vi "Lab Panel V5.29.vi"() -> ()   [LabVIEW 2013] (continued)
                    n2198 = Multiply(x=w3863, y=w3857) -> (x*y=w3850:dbl)
                    n2199 = Multiply(x=w3862, y=w3856) -> (x*y=w3849:dbl)
                    n2200 = Multiply(x=w3861, y=w3855) -> (x*y=w3848:dbl)
                    n2201 = Multiply(x=w3860, y=w3854) -> (x*y=w3846:dbl)
                    n2202 = Multiply(x=w3859, y=w3853) -> (x*y=w3845:dbl)
                    n2203 = Multiply(x=w3858, y=w3852) -> (x*y=w3844:dbl)
                    n2204 = local read "SIG LAB02-1"() -> (w3851:T2)
                    n2205 = local read "SIG LAB02-2"() -> (w3847:T2)
                    n2206 = Bundle By Name(cluster=w3851, "AMPS"=w3850, "VOLTS"=w3849, "PF"=w3848) -> (w3843:T2)
                    n2207 = Bundle By Name(cluster=w3847, "AMPS"=w3846, "VOLTS"=w3845, "PF"=w3844) -> (w3842:T2)
                    n2208 = global write "Global display 1.vi" "SIG LAB02-1"(w3843) -> ()
                    n2209 = local write "SIG LAB02-2"(w3842) -> ()
                    n2210 = global write "Global display 1.vi" "SIG LAB02-2"(w3842) -> ()
                    n2211 = local write "SIG LAB02-1"(w3843) -> ()
                  }
                  frame #4 {
                    n2212 = Unbundle By Name(w3895) -> ("OFF amps"=w3891:dbl, "VOLTS"=w3890:dbl, "PF"=w3889:dbl, "OFF amps"=w3888:dbl, "VOLTS"=w3887:dbl, "PF"=w3886:dbl)
                    n2213 = case shown="True" w3894 {
                      tunnel: [w3896 w3897] -> w3892
                      tunnel: w3893 -> [_ w3897]
                      frame False {
                        n2214 = local read "CAL LAB03"() -> (w3896:T14)
                      }
                      frame True {
                      }
                    }
                    n2215 = Unbundle By Name(w3892) -> ("1  (A) cal"=w3885:dbl, "1 (V) cal"=w3884:dbl, "1 (PF) cal"=w3883:dbl, "2 (A) cal"=w3882:dbl, "2 (V) cal"=w3881:dbl, "2 (PF) cal"=w3880:dbl)  [unwired: 4 out]
                    n2216 = Multiply(x=w3891, y=w3885) -> (x*y=w3878:dbl)
                    n2217 = Multiply(x=w3890, y=w3884) -> (x*y=w3872:dbl)
                    n2218 = Multiply(x=w3889, y=w3883) -> (x*y=w3877:dbl)
                    n2219 = Multiply(x=w3888, y=w3882) -> (x*y=w3875:dbl)
                    n2220 = Multiply(x=w3887, y=w3881) -> (x*y=w3874:dbl)
                    n2221 = Multiply(x=w3886, y=w3880) -> (x*y=w3873:dbl)
                    n2222 = local read "SIG LAB03-1"() -> (w3879:T2)
                    n2223 = local read "SIG LAB03-2"() -> (w3876:T2)
                    n2224 = Bundle By Name(cluster=w3879, "AMPS"=w3878, "VOLTS"=w3872, "PF"=w3877) -> (w3871:T2)
                    n2225 = Bundle By Name(cluster=w3876, "AMPS"=w3875, "VOLTS"=w3874, "PF"=w3873) -> (w3870:T2)
                    n2226 = global write "Global display 1.vi" "SIG LAB03-1"(w3871) -> ()
                    n2227 = global write "Global display 1.vi" "SIG LAB03-2"(w3870) -> ()
                    n2228 = local write "SIG LAB03-2"(w3870) -> ()
                    n2229 = local write "SIG LAB03-1"(w3871) -> ()
                  }
                  frame #5 {
                    n2230 = case shown="False" w3922 {
                      tunnel: [w3924 w3925] -> w3920
                      tunnel: w3921 -> [_ w3925]
                      frame False {
                        n2231 = local read "CAL LAB04"() -> (w3924:T14)
                      }
                      frame True {
                      }
                    }
                    n2232 = Unbundle By Name(w3923) -> ("OFF amps"=w3919:dbl, "VOLTS"=w3918:dbl, "PF"=w3917:dbl, "OFF amps"=w3916:dbl, "VOLTS"=w3915:dbl, "PF"=w3914:dbl)
                    n2233 = Unbundle By Name(w3920) -> ("1  (A) cal"=w3913:dbl, "1 (V) cal"=w3912:dbl, "1 (PF) cal"=w3911:dbl, "2 (A) cal"=w3910:dbl, "2 (V) cal"=w3909:dbl, "2 (PF) cal"=w3908:dbl)  [unwired: 4 out]
                    n2234 = Multiply(x=w3919, y=w3913) -> (x*y=w3906:dbl)
                    n2235 = Multiply(x=w3918, y=w3912) -> (x*y=w3905:dbl)
                    n2236 = Multiply(x=w3917, y=w3911) -> (x*y=w3904:dbl)
                    n2237 = Multiply(x=w3916, y=w3910) -> (x*y=w3902:dbl)
                    n2238 = Multiply(x=w3915, y=w3909) -> (x*y=w3901:dbl)
                    n2239 = Multiply(x=w3914, y=w3908) -> (x*y=w3900:dbl)
                    n2240 = local read "SIG LAB04-1"() -> (w3907:T2)
                    n2241 = local read "SIG LAB04-2"() -> (w3903:T2)
                    n2242 = Bundle By Name(cluster=w3907, "AMPS"=w3906, "VOLTS"=w3905, "PF"=w3904) -> (w3899:T2)
                    n2243 = Bundle By Name(cluster=w3903, "AMPS"=w3902, "VOLTS"=w3901, "PF"=w3900) -> (w3898:T2)
                    n2244 = global write "Global display 1.vi" "SIG LAB04-2"(w3898) -> ()
                    n2245 = global write "Global display 1.vi" "SIG LAB04-1"(w3899) -> ()
                    n2246 = local write "SIG LAB04-2"(w3898) -> ()
                    n2247 = local write "SIG LAB04-1"(w3899) -> ()
                  }
                  frame #6 {
                    n2248 = Unbundle By Name(w3951) -> ("OFF amps"=w3947:dbl, "VOLTS"=w3928:dbl, "PF"=w3946:dbl, "OFF amps"=w3945:dbl, "VOLTS"=w3944:dbl, "PF"=w3943:dbl)
                    n2249 = case shown="False" w3950 {
                      tunnel: [w3952 w3953] -> w3948
                      tunnel: w3949 -> [_ w3953]
                      frame False {
                        n2250 = local read "CAL LAB05"() -> (w3952:T14)
                      }
                      frame True {
                      }
                    }
                    n2251 = Unbundle By Name(w3948) -> ("1  (A) cal"=w3942:dbl, "1 (V) cal"=w3941:dbl, "1 (PF) cal"=w3940:dbl, "2 (A) cal"=w3939:dbl, "2 (V) cal"=w3938:dbl, "2 (PF) cal"=w3937:dbl)  [unwired: 4 out]
                    n2252 = Multiply(x=w3947, y=w3942) -> (x*y=w3935:dbl)
                    n2253 = Multiply(x=w3928, y=w3941) -> (x*y=w3934:dbl)
                    n2254 = Multiply(x=w3946, y=w3940) -> (x*y=w3933:dbl)
                    n2255 = Multiply(x=w3945, y=w3939) -> (x*y=w3931:dbl)
                    n2256 = Multiply(x=w3944, y=w3938) -> (x*y=w3930:dbl)
                    n2257 = Multiply(x=w3943, y=w3937) -> (x*y=w3929:dbl)
                    n2258 = local read "SIG LAB05-1"() -> (w3936:T2)
                    n2259 = local read "SIG LAB05-2"() -> (w3932:T2)
                    n2260 = Bundle By Name(cluster=w3936, "AMPS"=w3935, "VOLTS"=w3934, "PF"=w3933) -> (w3927:T2)
                    n2261 = Bundle By Name(cluster=w3932, "AMPS"=w3931, "VOLTS"=w3930, "PF"=w3929) -> (w3926:T2)
                    n2262 = global write "Global display 1.vi" "SIG LAB05-1"(w3927) -> ()
                    n2263 = global write "Global display 1.vi" "SIG LAB05-2"(w3926) -> ()
                    n2264 = local write "SIG LAB05-2"(w3926) -> ()
                    n2265 = local write "SIG LAB05-1"(w3927) -> ()
                  }
                  frame #7 {
                    n2266 = case shown="False" w3954 {
                      tunnel: w3956 -> [w3961 _]
                      tunnel: w3955 -> [w3960 _]
                      frame False {
                        # "update ambient referance temperature"
                        n2267 = case shown="True" w3961 {
                          tunnel: [w3963 100.0] -> w3962
                          frame False {
                            n2268 = local read "TEMP REF cal"() -> (w3963:dbl)
                          }
                          frame True {
                          }
                        }
                        n2269 = disable-structure shown="Disabled" {
                          frame Disabled {
                            n2270 = local read "Temp read loop"() -> ()  [unwired: 1 out]
                          }
                          frame Enabled {
                          }
                        }
                        n2271 = Multiply(x=w3962, y=w3960) -> (x*y=w3959:dbl)
                        n2272 = Subtract(x=w3959, y=272) -> (x-y=w3957:dbl)
                        "Amb Tp" <- w3957
                        n2273 = local write "Ref deg C"(w3957) -> ()
                        "deg C (volts)" <- w3960
                      }
                      frame True {
                      }
                    }
                  }
                }
              }
            }
          }
          frame #14 {
            # "save test data to file during testing"
            n2274 = local read "on loops"() -> (w3984:dbl)
            n2275 = Get Date/Time In Seconds() -> (seconds since 1Jan1904=w3965:timestamp)
            "File Time Stamp" <- w3965
            n2276 = local read "jig cycle"() -> (w3981:dbl)
            n2277 = Format Date/Time String(time format string (%c)="%H:%M%:%S", seconds (now)=w3965) -> (date/time string=w3969:string)  [unwired: 1 in]
            n2278 = Add(x=w3984, y=4) -> (x+y=w3982:dbl)
            n2279 = Build Array(w3969) -> (w3968:string[])
            n2280 = Equal?(x=w3981, y=3) -> (x = y?=w3967:bool)
            n2281 = Equal?(x=w3981, y=w3982) -> (x = y?=w3966:bool)
            n2282 = stacked-sequence {
              tunnel: w3980 -> [w3990 _ _ _ _ _ _ _ _ _]
              tunnel: w3979 -> [_ w4066 _ _ _ _ _ _ _ _]
              tunnel: w3978 -> [_ _ w4146 _ _ _ _ _ _ _]
              tunnel: w3977 -> [_ _ _ w4226 _ _ _ _ _ _]
              tunnel: w3976 -> [_ _ _ _ w4306 _ _ _ _ _]
              tunnel: w3975 -> [_ _ _ _ _ w4386 _ _ _ _]
              tunnel: w3974 -> [_ _ _ _ _ _ w4466 _ _ _]
              tunnel: w3973 -> [_ _ _ _ _ _ _ w4546 _ _]
              tunnel: w3972 -> [_ _ _ _ _ _ _ _ w4626 _]
              tunnel: w3971 -> [_ _ _ _ _ _ _ _ _ w4706]
              tunnel: w3968 -> [w3989 w4070 w4150 w4230 w4310 w4390 w4470 w4550 w4630 w4710]
              tunnel: w3967 -> [w3988 w4069 w4149 w4229 w4309 w4389 w4469 w4549 w4629 w4709]
              tunnel: w3966 -> [w3987 w4068 w4148 w4228 w4308 w4388 w4468 w4548 w4628 w4708]
              tunnel: w3965 -> [w3986 w4067 w4147 w4227 w4307 w4387 w4467 w4547 w4627 w4707]
              frame #0 {
                n2283 = case shown="True" w3990 {
                  tunnel: w3989 -> [_ w3995]
                  tunnel: w3988 -> [_ w3994]
                  tunnel: w3987 -> [_ w3992]
                  tunnel: w3986 -> [_ w3991]
                  frame False {
                  }
                  frame True {
                    n2284 = local read "DISP LAB01-1"() -> (w3996:T4)
                    n2285 = local read "SIG LAB01-1"() -> (w3997:T2)
                    n2286 = local read "ON L01-1"() -> (w3993:cluster{"amps":dbl, "volts":dbl, "pf":dbl})
                    n2287 = Unbundle(w3997) -> ("AMPS"=w4003:dbl, "VOLTS"=w4001:dbl, "PF"=w4000:dbl, "Tmp Live"=w3999:dbl, "Tmp Neut"=w4002:dbl)
                    n2288 = Unbundle(w3996) -> ("CYCLE"=w3998:dbl)  [unwired: 2 out]
                    n2289 = stacked-sequence {
                      tunnel: w4003 -> [w4007 w4026]
                      tunnel: w4002 -> [_ w4025]
                      tunnel: w4001 -> [w4006 w4024]
                      tunnel: w4000 -> [w4005 w4023]
                      tunnel: w3999 -> [_ w4022]
                      tunnel: w3998 -> [_ w4021]
                      tunnel: w3995 -> [_ w4020]
                      tunnel: w3994 -> [w4008 _]
                      tunnel: w3993 -> [w4004 w4018]
                      tunnel: w3992 -> [_ w4019]
                      tunnel: w3991 -> [_ w4014]
                      frame #0 {
                        n2290 = case shown="True" w4008 {
                          tunnel: w4007 -> [_ w4013]
                          tunnel: w4006 -> [_ w4012]
                          tunnel: w4005 -> [_ w4011]
                          tunnel: w4004 -> [_ w4009]
                          frame False {
                          }
                          frame True {
                            n2291 = Bundle(cluster=w4009, "amps"=w4013, "volts"=w4012, "pf"=w4011) -> (w4010:cluster{"amps":dbl, "volts":dbl, "pf":dbl})
                            n2292 = local write "ON L01-1"(w4010) -> ()
                          }
                        }
                      }
                      frame #1 {
                        n2293 = Unbundle(w4018) -> ("amps"=w4017:dbl, "volts"=w4016:dbl, "pf"=w4015:dbl)
                        n2294 = case shown="True" w4019 {
                          tunnel: w4026 -> [_ w4027]
                          tunnel: w4025 -> [_ w4065]
                          tunnel: w4024 -> [_ _]
                          tunnel: w4023 -> [_ _]
                          tunnel: w4022 -> [_ w4064]
                          tunnel: w4021 -> [_ w4063]
                          tunnel: w4020 -> [_ w4031]
                          tunnel: w4017 -> [_ w4028]
                          tunnel: w4016 -> [_ w4060]
                          tunnel: w4015 -> [_ w4059]
                          tunnel: w4014 -> [_ w4029]
                          frame False {
                          }
                          frame True {
                            n2295 = local read "TDMS LAB01-1"() -> (w4062:refnum<k34>)
                            n2296 = Build Array(w4060) -> (w4056:dbl[])
                            n2297 = Build Array(w4059) -> (w4055:dbl[])
                            n2298 = Build Array(w4064) -> (w4054:dbl[])
                            n2299 = Build Array(w4065) -> (w4053:dbl[])
                            n2300 = Build Array(w4028) -> (w4058:dbl[])
                            n2301 = Build Array(w4027) -> (w4057:dbl[])
                            n2302 = Build Array(w4063) -> (w4052:dbl[])
                            n2303 = Build Array("AMPS ON", "AMPS OFF", "VOLTS", "PF", "TEMP Live", "TEMP Neut", "CYCLE") -> (w4036:string[])
                            n2304 = Bundle By Name("Y"=w4058, "t0"=w4029) -> (w4051:waveform(dbl))  [unwired: 1 in]
                            n2305 = Bundle By Name("Y"=w4057, "t0"=w4029) -> (w4050:waveform(dbl))  [unwired: 1 in]
                            n2306 = Bundle By Name("Y"=w4056, "t0"=w4029) -> (w4049:waveform(dbl))  [unwired: 1 in]
                            n2307 = Bundle By Name("Y"=w4055, "t0"=w4029) -> (w4048:waveform(dbl))  [unwired: 1 in]
                            n2308 = Bundle By Name("Y"=w4054, "t0"=w4029) -> (w4047:waveform(dbl))  [unwired: 1 in]
                            n2309 = Bundle By Name("Y"=w4053, "t0"=w4029) -> (w4046:waveform(dbl))  [unwired: 1 in]
                            n2310 = Bundle By Name("Y"=w4052, "t0"=w4029) -> (w4045:waveform(dbl))  [unwired: 1 in]
                            n2311 = Build Array(w4051, w4050, w4049, w4048, w4047, w4046, w4045) -> (w4044:waveform(dbl)[])
                            n2312 = TDMS Write(0:w4062, 5:"TEST VALUES", 7:w4036, 9:w4044) -> (4:w4035:refnum<k34>, 6:w4034:string, 15:w4033:errorcluster)  [unwired: 2 in, 1 out]
                            n2313 = TDMS Write(0:w4035, 5:w4034, 7:"TIME", 9:w4031, 11:w4033) -> (15:w4030:errorcluster)  [unwired: 1 in, 3 out]
                            n2314 = local write "data file error"(w4030) -> ()
                          }
                        }
                      }
                    }
                  }
                }
              }
              frame #1 {
                n2315 = case shown="True" w4066 {
                  tunnel: w4070 -> [_ w4075]
                  tunnel: w4069 -> [_ w4074]
                  tunnel: w4068 -> [_ w4072]
                  tunnel: w4067 -> [_ w4071]
                  frame False {
                  }
                  frame True {
                    n2316 = local read "DISP LAB01-2"() -> (w4076:T4)
                    n2317 = local read "SIG LAB01-2"() -> (w4077:T2)
                    n2318 = local read "ON L01-2"() -> (w4073:cluster{"amps":dbl, "volts":dbl, "pf":dbl})
                    n2319 = Unbundle(w4077) -> ("AMPS"=w4083:dbl, "VOLTS"=w4081:dbl, "PF"=w4080:dbl, "Tmp Live"=w4079:dbl, "Tmp Neut"=w4082:dbl)
                    n2320 = Unbundle(w4076) -> ("CYCLE"=w4078:dbl)  [unwired: 2 out]
                    n2321 = stacked-sequence {
                      tunnel: w4083 -> [w4087 w4106]
                      tunnel: w4082 -> [_ w4105]
                      tunnel: w4081 -> [w4086 w4104]
                      tunnel: w4080 -> [w4085 w4103]
                      tunnel: w4079 -> [_ w4102]
                      tunnel: w4078 -> [_ w4101]
                      tunnel: w4075 -> [_ w4100]
                      tunnel: w4074 -> [w4088 _]
                      tunnel: w4073 -> [w4084 w4098]
                      tunnel: w4072 -> [_ w4099]
                      tunnel: w4071 -> [_ w4094]
                      frame #0 {
                        n2322 = case shown="True" w4088 {
                          tunnel: w4087 -> [_ w4093]
                          tunnel: w4086 -> [_ w4092]
                          tunnel: w4085 -> [_ w4091]
                          tunnel: w4084 -> [_ w4089]
                          frame False {
                          }
                          frame True {
                            n2323 = Bundle(cluster=w4089, "amps"=w4093, "volts"=w4092, "pf"=w4091) -> (w4090:cluster{"amps":dbl, "volts":dbl, "pf":dbl})
                            n2324 = local write "ON L01-2"(w4090) -> ()
                          }
                        }
                      }
                      frame #1 {
                        n2325 = Unbundle(w4098) -> ("amps"=w4097:dbl, "volts"=w4096:dbl, "pf"=w4095:dbl)
                        n2326 = case shown="True" w4099 {
                          tunnel: w4106 -> [_ w4138]
                          tunnel: w4105 -> [_ w4145]
                          tunnel: w4104 -> [_ _]
                          tunnel: w4103 -> [_ _]
                          tunnel: w4102 -> [_ w4144]
                          tunnel: w4101 -> [_ w4143]
                          tunnel: w4100 -> [_ w4108]
                          tunnel: w4097 -> [_ w4140]
                          tunnel: w4096 -> [_ w4139]
                          tunnel: w4095 -> [_ w4137]
                          tunnel: w4094 -> [_ w4129]
                          frame False {
                          }
                          frame True {
                            n2327 = local read "TDMS LAB01-2"() -> (w4142:refnum<k34>)
                            n2328 = Build Array(w4139) -> (w4134:dbl[])
                            n2329 = Build Array(w4137) -> (w4133:dbl[])
                            n2330 = Build Array(w4144) -> (w4132:dbl[])
                            n2331 = Build Array(w4145) -> (w4131:dbl[])
                            n2332 = Build Array(w4140) -> (w4136:dbl[])
                            n2333 = Build Array(w4138) -> (w4135:dbl[])
                            n2334 = Build Array(w4143) -> (w4130:dbl[])
                            n2335 = Build Array("AMPS ON", "AMPS OFF", "VOLTS", "PF", "TEMP Live", "TEMP Neut", "CYCLE") -> (w4113:string[])
                            n2336 = Bundle By Name("Y"=w4136, "t0"=w4129) -> (w4128:waveform(dbl))  [unwired: 1 in]
                            n2337 = Bundle By Name("Y"=w4135, "t0"=w4129) -> (w4127:waveform(dbl))  [unwired: 1 in]
                            n2338 = Bundle By Name("Y"=w4134, "t0"=w4129) -> (w4126:waveform(dbl))  [unwired: 1 in]
                            n2339 = Bundle By Name("Y"=w4133, "t0"=w4129) -> (w4125:waveform(dbl))  [unwired: 1 in]
                            n2340 = Bundle By Name("Y"=w4132, "t0"=w4129) -> (w4124:waveform(dbl))  [unwired: 1 in]
                            n2341 = Bundle By Name("Y"=w4131, "t0"=w4129) -> (w4123:waveform(dbl))  [unwired: 1 in]
                            n2342 = Bundle By Name("Y"=w4130, "t0"=w4129) -> (w4122:waveform(dbl))  [unwired: 1 in]
                            n2343 = Build Array(w4128, w4127, w4126, w4125, w4124, w4123, w4122) -> (w4121:waveform(dbl)[])
                            n2344 = TDMS Write(0:w4142, 5:"TEST VALUES", 7:w4113, 9:w4121) -> (4:w4112:refnum<k34>, 6:w4111:string, 15:w4110:errorcluster)  [unwired: 2 in, 1 out]
                            n2345 = TDMS Write(0:w4112, 5:w4111, 7:"TIME", 9:w4108, 11:w4110) -> (15:w4107:errorcluster)  [unwired: 1 in, 3 out]
                            n2346 = local write "data file error"(w4107) -> ()
                          }
                        }
                      }
                    }
                  }
                }
              }
              frame #2 {
                n2347 = case shown="True" w4146 {
                  tunnel: w4150 -> [_ w4155]
                  tunnel: w4149 -> [_ w4154]
                  tunnel: w4148 -> [_ w4152]
                  tunnel: w4147 -> [_ w4151]
                  frame False {
                  }
                  frame True {
                    n2348 = local read "DISP LAB02-1"() -> (w4156:T4)
                    n2349 = local read "SIG LAB02-1"() -> (w4157:T2)
                    n2350 = local read "ON L02-1"() -> (w4153:cluster{"amps":dbl, "volts":dbl, "pf":dbl})
                    n2351 = Unbundle(w4157) -> ("AMPS"=w4163:dbl, "VOLTS"=w4161:dbl, "PF"=w4160:dbl, "Tmp Live"=w4159:dbl, "Tmp Neut"=w4162:dbl)
                    n2352 = Unbundle(w4156) -> ("CYCLE"=w4158:dbl)  [unwired: 2 out]
                    n2353 = stacked-sequence {
                      tunnel: w4163 -> [w4167 w4186]
                      tunnel: w4162 -> [_ w4185]
                      tunnel: w4161 -> [w4166 w4184]
                      tunnel: w4160 -> [w4165 w4183]
                      tunnel: w4159 -> [_ w4182]
                      tunnel: w4158 -> [_ w4181]
                      tunnel: w4155 -> [_ w4180]
                      tunnel: w4154 -> [w4168 _]
                      tunnel: w4153 -> [w4164 w4178]
                      tunnel: w4152 -> [_ w4179]
                      tunnel: w4151 -> [_ w4174]
                      frame #0 {
                        n2354 = case shown="True" w4168 {
                          tunnel: w4167 -> [_ w4173]
                          tunnel: w4166 -> [_ w4172]
                          tunnel: w4165 -> [_ w4171]
                          tunnel: w4164 -> [_ w4169]
                          frame False {
                          }
                          frame True {
                            n2355 = Bundle(cluster=w4169, "amps"=w4173, "volts"=w4172, "pf"=w4171) -> (w4170:cluster{"amps":dbl, "volts":dbl, "pf":dbl})
                            n2356 = local write "ON L02-1"(w4170) -> ()
                          }
                        }
                      }
                      frame #1 {
                        n2357 = Unbundle(w4178) -> ("amps"=w4177:dbl, "volts"=w4176:dbl, "pf"=w4175:dbl)
                        n2358 = case shown="True" w4179 {
                          tunnel: w4186 -> [_ w4218]
                          tunnel: w4185 -> [_ w4225]
                          tunnel: w4184 -> [_ _]
                          tunnel: w4183 -> [_ _]
                          tunnel: w4182 -> [_ w4224]
                          tunnel: w4181 -> [_ w4223]
                          tunnel: w4180 -> [_ w4188]
                          tunnel: w4177 -> [_ w4220]
                          tunnel: w4176 -> [_ w4219]
                          tunnel: w4175 -> [_ w4217]
                          tunnel: w4174 -> [_ w4209]
                          frame False {
                          }
                          frame True {
                            n2359 = local read "TDMS LAB02-1"() -> (w4222:refnum<k34>)
                            n2360 = Build Array(w4219) -> (w4214:dbl[])
                            n2361 = Build Array(w4217) -> (w4213:dbl[])
                            n2362 = Build Array(w4224) -> (w4212:dbl[])
                            n2363 = Build Array(w4225) -> (w4211:dbl[])
                            n2364 = Build Array(w4220) -> (w4216:dbl[])
                            n2365 = Build Array(w4218) -> (w4215:dbl[])
                            n2366 = Build Array(w4223) -> (w4210:dbl[])
                            n2367 = Build Array("AMPS ON", "AMPS OFF", "VOLTS", "PF", "TEMP Live", "TEMP Neut", "CYCLE") -> (w4193:string[])
                            n2368 = Bundle By Name("Y"=w4216, "t0"=w4209) -> (w4208:waveform(dbl))  [unwired: 1 in]
                            n2369 = Bundle By Name("Y"=w4215, "t0"=w4209) -> (w4207:waveform(dbl))  [unwired: 1 in]
                            n2370 = Bundle By Name("Y"=w4214, "t0"=w4209) -> (w4206:waveform(dbl))  [unwired: 1 in]
                            n2371 = Bundle By Name("Y"=w4213, "t0"=w4209) -> (w4205:waveform(dbl))  [unwired: 1 in]
                            n2372 = Bundle By Name("Y"=w4212, "t0"=w4209) -> (w4204:waveform(dbl))  [unwired: 1 in]
                            n2373 = Bundle By Name("Y"=w4211, "t0"=w4209) -> (w4203:waveform(dbl))  [unwired: 1 in]
                            n2374 = Bundle By Name("Y"=w4210, "t0"=w4209) -> (w4202:waveform(dbl))  [unwired: 1 in]
                            n2375 = Build Array(w4208, w4207, w4206, w4205, w4204, w4203, w4202) -> (w4201:waveform(dbl)[])
                            n2376 = TDMS Write(0:w4222, 5:"TEST VALUES", 7:w4193, 9:w4201) -> (4:w4192:refnum<k34>, 6:w4191:string, 15:w4190:errorcluster)  [unwired: 2 in, 1 out]
                            n2377 = TDMS Write(0:w4192, 5:w4191, 7:"TIME", 9:w4188, 11:w4190) -> (15:w4187:errorcluster)  [unwired: 1 in, 3 out]
                            n2378 = local write "data file error"(w4187) -> ()
                          }
                        }
                      }
                    }
                  }
                }
              }
              frame #3 {
                n2379 = case shown="True" w4226 {
                  tunnel: w4230 -> [_ w4235]
                  tunnel: w4229 -> [_ w4234]
                  tunnel: w4228 -> [_ w4232]
                  tunnel: w4227 -> [_ w4231]
                  frame False {
                  }
                  frame True {
                    n2380 = local read "DISP LAB02-2"() -> (w4236:T4)
                    n2381 = local read "SIG LAB02-2"() -> (w4237:T2)
                    n2382 = local read "ON L02-2"() -> (w4233:cluster{"amps":dbl, "volts":dbl, "pf":dbl})
                    n2383 = Unbundle(w4237) -> ("AMPS"=w4243:dbl, "VOLTS"=w4241:dbl, "PF"=w4240:dbl, "Tmp Live"=w4239:dbl, "Tmp Neut"=w4242:dbl)
                    n2384 = Unbundle(w4236) -> ("CYCLE"=w4238:dbl)  [unwired: 2 out]
                    n2385 = stacked-sequence {
                      tunnel: w4243 -> [w4247 w4266]
                      tunnel: w4242 -> [_ w4265]
                      tunnel: w4241 -> [w4246 w4264]
                      tunnel: w4240 -> [w4245 w4263]
                      tunnel: w4239 -> [_ w4262]
                      tunnel: w4238 -> [_ w4261]
                      tunnel: w4235 -> [_ w4260]
                      tunnel: w4234 -> [w4248 _]
                      tunnel: w4233 -> [w4244 w4258]
                      tunnel: w4232 -> [_ w4259]
                      tunnel: w4231 -> [_ w4254]
                      frame #0 {
                        n2386 = case shown="True" w4248 {
                          tunnel: w4247 -> [_ w4253]
                          tunnel: w4246 -> [_ w4252]
                          tunnel: w4245 -> [_ w4251]
                          tunnel: w4244 -> [_ w4249]
                          frame False {
                          }
                          frame True {
                            n2387 = Bundle(cluster=w4249, "amps"=w4253, "volts"=w4252, "pf"=w4251) -> (w4250:cluster{"amps":dbl, "volts":dbl, "pf":dbl})
                            n2388 = local write "ON L02-2"(w4250) -> ()
                          }
                        }
                      }
                      frame #1 {
                        n2389 = Unbundle(w4258) -> ("amps"=w4257:dbl, "volts"=w4256:dbl, "pf"=w4255:dbl)
                        n2390 = case shown="True" w4259 {
                          tunnel: w4266 -> [_ w4298]
                          tunnel: w4265 -> [_ w4305]
                          tunnel: w4264 -> [_ _]
                          tunnel: w4263 -> [_ _]
                          tunnel: w4262 -> [_ w4304]
                          tunnel: w4261 -> [_ w4303]
                          tunnel: w4260 -> [_ w4268]
                          tunnel: w4257 -> [_ w4300]
                          tunnel: w4256 -> [_ w4299]
                          tunnel: w4255 -> [_ w4297]
                          tunnel: w4254 -> [_ w4289]
                          frame False {
                          }
                          frame True {
                            n2391 = local read "TDMS LAB02-2"() -> (w4302:refnum<k34>)
                            n2392 = Build Array(w4299) -> (w4294:dbl[])
                            n2393 = Build Array(w4297) -> (w4293:dbl[])
                            n2394 = Build Array(w4304) -> (w4292:dbl[])
                            n2395 = Build Array(w4305) -> (w4291:dbl[])
                            n2396 = Build Array(w4300) -> (w4296:dbl[])
                            n2397 = Build Array(w4298) -> (w4295:dbl[])
                            n2398 = Build Array(w4303) -> (w4290:dbl[])
                            n2399 = Build Array("AMPS ON", "AMPS OFF", "VOLTS", "PF", "TEMP Live", "TEMP Neut", "CYCLE") -> (w4273:string[])
                            n2400 = Bundle By Name("Y"=w4296, "t0"=w4289) -> (w4288:waveform(dbl))  [unwired: 1 in]
                            n2401 = Bundle By Name("Y"=w4295, "t0"=w4289) -> (w4287:waveform(dbl))  [unwired: 1 in]
                            n2402 = Bundle By Name("Y"=w4294, "t0"=w4289) -> (w4286:waveform(dbl))  [unwired: 1 in]
                            n2403 = Bundle By Name("Y"=w4293, "t0"=w4289) -> (w4285:waveform(dbl))  [unwired: 1 in]
                            n2404 = Bundle By Name("Y"=w4292, "t0"=w4289) -> (w4284:waveform(dbl))  [unwired: 1 in]
                            n2405 = Bundle By Name("Y"=w4291, "t0"=w4289) -> (w4283:waveform(dbl))  [unwired: 1 in]
                            n2406 = Bundle By Name("Y"=w4290, "t0"=w4289) -> (w4282:waveform(dbl))  [unwired: 1 in]
                            n2407 = Build Array(w4288, w4287, w4286, w4285, w4284, w4283, w4282) -> (w4281:waveform(dbl)[])
                            n2408 = TDMS Write(0:w4302, 5:"TEST VALUES", 7:w4273, 9:w4281) -> (4:w4272:refnum<k34>, 6:w4271:string, 15:w4270:errorcluster)  [unwired: 2 in, 1 out]
                            n2409 = TDMS Write(0:w4272, 5:w4271, 7:"TIME", 9:w4268, 11:w4270) -> (15:w4267:errorcluster)  [unwired: 1 in, 3 out]
                            n2410 = local write "data file error"(w4267) -> ()
                          }
                        }
                      }
                    }
                  }
                }
              }
              frame #4 {
                n2411 = case shown="True" w4306 {
                  tunnel: w4310 -> [_ w4315]
                  tunnel: w4309 -> [_ w4314]
                  tunnel: w4308 -> [_ w4312]
                  tunnel: w4307 -> [_ w4311]
                  frame False {
                  }
                  frame True {
                    n2412 = local read "DISP LAB03-1"() -> (w4316:T4)
                    n2413 = local read "SIG LAB03-1"() -> (w4317:T2)
                    n2414 = local read "ON L03-1"() -> (w4313:cluster{"amps":dbl, "volts":dbl, "pf":dbl})
                    n2415 = Unbundle(w4317) -> ("AMPS"=w4323:dbl, "VOLTS"=w4321:dbl, "PF"=w4320:dbl, "Tmp Live"=w4319:dbl, "Tmp Neut"=w4322:dbl)
                    n2416 = Unbundle(w4316) -> ("CYCLE"=w4318:dbl)  [unwired: 2 out]
                    n2417 = stacked-sequence {
                      tunnel: w4323 -> [w4327 w4346]
                      tunnel: w4322 -> [_ w4345]
                      tunnel: w4321 -> [w4326 w4344]
                      tunnel: w4320 -> [w4325 w4343]
                      tunnel: w4319 -> [_ w4342]
                      tunnel: w4318 -> [_ w4341]
                      tunnel: w4315 -> [_ w4340]
                      tunnel: w4314 -> [w4328 _]
                      tunnel: w4313 -> [w4324 w4338]
                      tunnel: w4312 -> [_ w4339]
                      tunnel: w4311 -> [_ w4334]
                      frame #0 {
                        n2418 = case shown="True" w4328 {
                          tunnel: w4327 -> [_ w4333]
                          tunnel: w4326 -> [_ w4332]
                          tunnel: w4325 -> [_ w4331]
                          tunnel: w4324 -> [_ w4329]
                          frame False {
                          }
                          frame True {
                            n2419 = Bundle(cluster=w4329, "amps"=w4333, "volts"=w4332, "pf"=w4331) -> (w4330:cluster{"amps":dbl, "volts":dbl, "pf":dbl})
                            n2420 = local write "ON L03-1"(w4330) -> ()
                          }
                        }
                      }
                      frame #1 {
                        n2421 = Unbundle(w4338) -> ("amps"=w4337:dbl, "volts"=w4336:dbl, "pf"=w4335:dbl)
                        n2422 = case shown="True" w4339 {
                          tunnel: w4346 -> [_ w4378]
                          tunnel: w4345 -> [_ w4385]
                          tunnel: w4344 -> [_ _]
                          tunnel: w4343 -> [_ _]
                          tunnel: w4342 -> [_ w4384]
                          tunnel: w4341 -> [_ w4383]
                          tunnel: w4340 -> [_ w4348]
                          tunnel: w4337 -> [_ w4380]
                          tunnel: w4336 -> [_ w4379]
                          tunnel: w4335 -> [_ w4377]
                          tunnel: w4334 -> [_ w4369]
                          frame False {
                          }
                          frame True {
                            n2423 = local read "TDMS LAB03-1"() -> (w4382:refnum<k34>)
                            n2424 = Build Array(w4379) -> (w4374:dbl[])
                            n2425 = Build Array(w4377) -> (w4373:dbl[])
                            n2426 = Build Array(w4384) -> (w4372:dbl[])
                            n2427 = Build Array(w4385) -> (w4371:dbl[])
                            n2428 = Build Array(w4380) -> (w4376:dbl[])
                            n2429 = Build Array(w4378) -> (w4375:dbl[])
                            n2430 = Build Array(w4383) -> (w4370:dbl[])
                            n2431 = Build Array("AMPS ON", "AMPS OFF", "VOLTS", "PF", "TEMP Live", "TEMP Neut", "CYCLE") -> (w4353:string[])
                            n2432 = Bundle By Name("Y"=w4376, "t0"=w4369) -> (w4368:waveform(dbl))  [unwired: 1 in]
                            n2433 = Bundle By Name("Y"=w4375, "t0"=w4369) -> (w4367:waveform(dbl))  [unwired: 1 in]
                            n2434 = Bundle By Name("Y"=w4374, "t0"=w4369) -> (w4366:waveform(dbl))  [unwired: 1 in]
                            n2435 = Bundle By Name("Y"=w4373, "t0"=w4369) -> (w4365:waveform(dbl))  [unwired: 1 in]
                            n2436 = Bundle By Name("Y"=w4372, "t0"=w4369) -> (w4364:waveform(dbl))  [unwired: 1 in]
                            n2437 = Bundle By Name("Y"=w4371, "t0"=w4369) -> (w4363:waveform(dbl))  [unwired: 1 in]
                            n2438 = Bundle By Name("Y"=w4370, "t0"=w4369) -> (w4362:waveform(dbl))  [unwired: 1 in]
                            n2439 = Build Array(w4368, w4367, w4366, w4365, w4364, w4363, w4362) -> (w4361:waveform(dbl)[])
                            n2440 = TDMS Write(0:w4382, 5:"TEST VALUES", 7:w4353, 9:w4361) -> (4:w4352:refnum<k34>, 6:w4351:string, 15:w4350:errorcluster)  [unwired: 2 in, 1 out]
                            n2441 = TDMS Write(0:w4352, 5:w4351, 7:"TIME", 9:w4348, 11:w4350) -> (15:w4347:errorcluster)  [unwired: 1 in, 3 out]
                            n2442 = local write "data file error"(w4347) -> ()
                          }
                        }
                      }
                    }
                  }
                }
              }
              frame #5 {
                n2443 = case shown="True" w4386 {
                  tunnel: w4390 -> [_ w4395]
                  tunnel: w4389 -> [_ w4394]
                  tunnel: w4388 -> [_ w4392]
                  tunnel: w4387 -> [_ w4391]
                  frame False {
                  }
                  frame True {
                    n2444 = local read "DISP LAB03-2"() -> (w4396:T4)
                    n2445 = local read "SIG LAB03-2"() -> (w4397:T2)
                    n2446 = local read "ON L03-2"() -> (w4393:cluster{"amps":dbl, "volts":dbl, "pf":dbl})
                    n2447 = Unbundle(w4397) -> ("AMPS"=w4403:dbl, "VOLTS"=w4401:dbl, "PF"=w4400:dbl, "Tmp Live"=w4399:dbl, "Tmp Neut"=w4402:dbl)
                    n2448 = Unbundle(w4396) -> ("CYCLE"=w4398:dbl)  [unwired: 2 out]
                    n2449 = stacked-sequence {
                      tunnel: w4403 -> [w4407 w4426]
                      tunnel: w4402 -> [_ w4425]
                      tunnel: w4401 -> [w4406 w4424]
                      tunnel: w4400 -> [w4405 w4423]
                      tunnel: w4399 -> [_ w4422]
                      tunnel: w4398 -> [_ w4421]
                      tunnel: w4395 -> [_ w4420]
                      tunnel: w4394 -> [w4408 _]
                      tunnel: w4393 -> [w4404 w4418]
                      tunnel: w4392 -> [_ w4419]
                      tunnel: w4391 -> [_ w4414]
                      frame #0 {
                        n2450 = case shown="True" w4408 {
                          tunnel: w4407 -> [_ w4413]
                          tunnel: w4406 -> [_ w4412]
                          tunnel: w4405 -> [_ w4411]
                          tunnel: w4404 -> [_ w4409]
                          frame False {
                          }
                          frame True {
                            n2451 = Bundle(cluster=w4409, "amps"=w4413, "volts"=w4412, "pf"=w4411) -> (w4410:cluster{"amps":dbl, "volts":dbl, "pf":dbl})
                            n2452 = local write "ON L03-2"(w4410) -> ()
                          }
                        }
                      }
                      frame #1 {
                        n2453 = Unbundle(w4418) -> ("amps"=w4417:dbl, "volts"=w4416:dbl, "pf"=w4415:dbl)
                        n2454 = case shown="True" w4419 {
                          tunnel: w4426 -> [_ w4458]
                          tunnel: w4425 -> [_ w4465]
                          tunnel: w4424 -> [_ _]
                          tunnel: w4423 -> [_ _]
                          tunnel: w4422 -> [_ w4464]
                          tunnel: w4421 -> [_ w4463]
                          tunnel: w4420 -> [_ w4428]
                          tunnel: w4417 -> [_ w4460]
                          tunnel: w4416 -> [_ w4459]
                          tunnel: w4415 -> [_ w4457]
                          tunnel: w4414 -> [_ w4449]
                          frame False {
                          }
                          frame True {
                            n2455 = local read "TDMS LAB03-2"() -> (w4462:refnum<k34>)
                            n2456 = Build Array(w4459) -> (w4454:dbl[])
                            n2457 = Build Array(w4457) -> (w4453:dbl[])
                            n2458 = Build Array(w4464) -> (w4452:dbl[])
                            n2459 = Build Array(w4465) -> (w4451:dbl[])
                            n2460 = Build Array(w4460) -> (w4456:dbl[])
                            n2461 = Build Array(w4458) -> (w4455:dbl[])
                            n2462 = Build Array(w4463) -> (w4450:dbl[])
                            n2463 = Build Array("AMPS ON", "AMPS OFF", "VOLTS", "PF", "TEMP Live", "TEMP Neut", "CYCLE") -> (w4433:string[])
                            n2464 = Bundle By Name("Y"=w4456, "t0"=w4449) -> (w4448:waveform(dbl))  [unwired: 1 in]
                            n2465 = Bundle By Name("Y"=w4455, "t0"=w4449) -> (w4447:waveform(dbl))  [unwired: 1 in]
                            n2466 = Bundle By Name("Y"=w4454, "t0"=w4449) -> (w4446:waveform(dbl))  [unwired: 1 in]
                            n2467 = Bundle By Name("Y"=w4453, "t0"=w4449) -> (w4445:waveform(dbl))  [unwired: 1 in]
                            n2468 = Bundle By Name("Y"=w4452, "t0"=w4449) -> (w4444:waveform(dbl))  [unwired: 1 in]
                            n2469 = Bundle By Name("Y"=w4451, "t0"=w4449) -> (w4443:waveform(dbl))  [unwired: 1 in]
                            n2470 = Bundle By Name("Y"=w4450, "t0"=w4449) -> (w4442:waveform(dbl))  [unwired: 1 in]
                            n2471 = Build Array(w4448, w4447, w4446, w4445, w4444, w4443, w4442) -> (w4441:waveform(dbl)[])
                            n2472 = TDMS Write(0:w4462, 5:"TEST VALUES", 7:w4433, 9:w4441) -> (4:w4432:refnum<k34>, 6:w4431:string, 15:w4430:errorcluster)  [unwired: 2 in, 1 out]
                            n2473 = TDMS Write(0:w4432, 5:w4431, 7:"TIME", 9:w4428, 11:w4430) -> (15:w4427:errorcluster)  [unwired: 1 in, 3 out]
                            n2474 = local write "data file error"(w4427) -> ()
                          }
                        }
                      }
                    }
                  }
                }
              }
              frame #6 {
                n2475 = case shown="True" w4466 {
                  tunnel: w4470 -> [_ w4475]
                  tunnel: w4469 -> [_ w4474]
                  tunnel: w4468 -> [_ w4472]
                  tunnel: w4467 -> [_ w4471]
                  frame False {
                  }
                  frame True {
                    n2476 = local read "DISP LAB04-1"() -> (w4476:T4)
                    n2477 = local read "SIG LAB04-1"() -> (w4477:T2)
                    n2478 = local read "ON L04-1"() -> (w4473:cluster{"amps":dbl, "volts":dbl, "pf":dbl})
                    n2479 = Unbundle(w4477) -> ("AMPS"=w4483:dbl, "VOLTS"=w4481:dbl, "PF"=w4480:dbl, "Tmp Live"=w4479:dbl, "Tmp Neut"=w4482:dbl)
                    n2480 = Unbundle(w4476) -> ("CYCLE"=w4478:dbl)  [unwired: 2 out]
                    n2481 = stacked-sequence {
                      tunnel: w4483 -> [w4487 w4506]
                      tunnel: w4482 -> [_ w4505]
                      tunnel: w4481 -> [w4486 w4504]
                      tunnel: w4480 -> [w4485 w4503]
                      tunnel: w4479 -> [_ w4502]
                      tunnel: w4478 -> [_ w4501]
                      tunnel: w4475 -> [_ w4500]
                      tunnel: w4474 -> [w4488 _]
                      tunnel: w4473 -> [w4484 w4498]
                      tunnel: w4472 -> [_ w4499]
                      tunnel: w4471 -> [_ w4494]
                      frame #0 {
                        n2482 = case shown="True" w4488 {
                          tunnel: w4487 -> [_ w4493]
                          tunnel: w4486 -> [_ w4492]
                          tunnel: w4485 -> [_ w4491]
                          tunnel: w4484 -> [_ w4489]
                          frame False {
                          }
                          frame True {
                            n2483 = Bundle(cluster=w4489, "amps"=w4493, "volts"=w4492, "pf"=w4491) -> (w4490:cluster{"amps":dbl, "volts":dbl, "pf":dbl})
                            n2484 = local write "ON L04-1"(w4490) -> ()
                          }
                        }
                      }
                      frame #1 {
                        n2485 = Unbundle(w4498) -> ("amps"=w4497:dbl, "volts"=w4496:dbl, "pf"=w4495:dbl)
                        n2486 = case shown="True" w4499 {
                          tunnel: w4506 -> [_ w4538]
                          tunnel: w4505 -> [_ w4545]
                          tunnel: w4504 -> [_ _]
                          tunnel: w4503 -> [_ _]
                          tunnel: w4502 -> [_ w4544]
                          tunnel: w4501 -> [_ w4543]
                          tunnel: w4500 -> [_ w4508]
                          tunnel: w4497 -> [_ w4540]
                          tunnel: w4496 -> [_ w4539]
                          tunnel: w4495 -> [_ w4537]
                          tunnel: w4494 -> [_ w4529]
                          frame False {
                          }
                          frame True {
                            n2487 = local read "TDMS LAB04-1"() -> (w4542:refnum<k34>)
                            n2488 = Build Array(w4539) -> (w4534:dbl[])
                            n2489 = Build Array(w4537) -> (w4533:dbl[])
                            n2490 = Build Array(w4544) -> (w4532:dbl[])
                            n2491 = Build Array(w4545) -> (w4531:dbl[])
                            n2492 = Build Array(w4540) -> (w4536:dbl[])
                            n2493 = Build Array(w4538) -> (w4535:dbl[])
                            n2494 = Build Array(w4543) -> (w4530:dbl[])
                            n2495 = Build Array("AMPS ON", "AMPS OFF", "VOLTS", "PF", "TEMP Live", "TEMP Neut", "CYCLE") -> (w4513:string[])
                            n2496 = Bundle By Name("Y"=w4536, "t0"=w4529) -> (w4528:waveform(dbl))  [unwired: 1 in]
                            n2497 = Bundle By Name("Y"=w4535, "t0"=w4529) -> (w4527:waveform(dbl))  [unwired: 1 in]
                            n2498 = Bundle By Name("Y"=w4534, "t0"=w4529) -> (w4526:waveform(dbl))  [unwired: 1 in]
                            n2499 = Bundle By Name("Y"=w4533, "t0"=w4529) -> (w4525:waveform(dbl))  [unwired: 1 in]
                            n2500 = Bundle By Name("Y"=w4532, "t0"=w4529) -> (w4524:waveform(dbl))  [unwired: 1 in]
                            n2501 = Bundle By Name("Y"=w4531, "t0"=w4529) -> (w4523:waveform(dbl))  [unwired: 1 in]
                            n2502 = Bundle By Name("Y"=w4530, "t0"=w4529) -> (w4522:waveform(dbl))  [unwired: 1 in]
                            n2503 = Build Array(w4528, w4527, w4526, w4525, w4524, w4523, w4522) -> (w4521:waveform(dbl)[])
                            n2504 = TDMS Write(0:w4542, 5:"TEST VALUES", 7:w4513, 9:w4521) -> (4:w4512:refnum<k34>, 6:w4511:string, 15:w4510:errorcluster)  [unwired: 2 in, 1 out]
                            n2505 = TDMS Write(0:w4512, 5:w4511, 7:"TIME", 9:w4508, 11:w4510) -> (15:w4507:errorcluster)  [unwired: 1 in, 3 out]
                            n2506 = local write "data file error"(w4507) -> ()
                          }
                        }
                      }
                    }
                  }
                }
              }
              frame #7 {
                n2507 = case shown="True" w4546 {
                  tunnel: w4550 -> [_ w4555]
                  tunnel: w4549 -> [_ w4554]
                  tunnel: w4548 -> [_ w4552]
                  tunnel: w4547 -> [_ w4551]
                  frame False {
                  }
                  frame True {
                    n2508 = local read "DISP LAB04-2"() -> (w4556:T4)
                    n2509 = local read "SIG LAB04-2"() -> (w4557:T2)
                    n2510 = local read "ON L04-2"() -> (w4553:cluster{"amps":dbl, "volts":dbl, "pf":dbl})
                    n2511 = Unbundle(w4557) -> ("AMPS"=w4563:dbl, "VOLTS"=w4561:dbl, "PF"=w4560:dbl, "Tmp Live"=w4559:dbl, "Tmp Neut"=w4562:dbl)
                    n2512 = Unbundle(w4556) -> ("CYCLE"=w4558:dbl)  [unwired: 2 out]
                    n2513 = stacked-sequence {
                      tunnel: w4563 -> [w4567 w4586]
                      tunnel: w4562 -> [_ w4585]
                      tunnel: w4561 -> [w4566 w4584]
                      tunnel: w4560 -> [w4565 w4583]
                      tunnel: w4559 -> [_ w4582]
                      tunnel: w4558 -> [_ w4581]
                      tunnel: w4555 -> [_ w4580]
                      tunnel: w4554 -> [w4568 _]
                      tunnel: w4553 -> [w4564 w4578]
                      tunnel: w4552 -> [_ w4579]
                      tunnel: w4551 -> [_ w4574]
                      frame #0 {
                        n2514 = case shown="True" w4568 {
                          tunnel: w4567 -> [_ w4573]
                          tunnel: w4566 -> [_ w4572]
                          tunnel: w4565 -> [_ w4571]
                          tunnel: w4564 -> [_ w4569]
                          frame False {
                          }
                          frame True {
                            n2515 = Bundle(cluster=w4569, "amps"=w4573, "volts"=w4572, "pf"=w4571) -> (w4570:cluster{"amps":dbl, "volts":dbl, "pf":dbl})
                            n2516 = local write "ON L04-2"(w4570) -> ()
                          }
                        }
                      }
                      frame #1 {
                        n2517 = Unbundle(w4578) -> ("amps"=w4577:dbl, "volts"=w4576:dbl, "pf"=w4575:dbl)
                        n2518 = case shown="True" w4579 {
                          tunnel: w4586 -> [_ w4618]
                          tunnel: w4585 -> [_ w4625]
                          tunnel: w4584 -> [_ _]
                          tunnel: w4583 -> [_ _]
                          tunnel: w4582 -> [_ w4624]
                          tunnel: w4581 -> [_ w4623]
                          tunnel: w4580 -> [_ w4588]
                          tunnel: w4577 -> [_ w4620]
                          tunnel: w4576 -> [_ w4619]
                          tunnel: w4575 -> [_ w4617]
                          tunnel: w4574 -> [_ w4609]
                          frame False {
                          }
                          frame True {
                            n2519 = local read "TDMS LAB04-2"() -> (w4622:refnum<k34>)
                            n2520 = Build Array(w4619) -> (w4614:dbl[])
                            n2521 = Build Array(w4617) -> (w4613:dbl[])
